vi "control.vi"() -> ()   [LabVIEW 2018]
uses:
  <vilib>/Analysis/Matrix/Datatypes/RealMatrix.ctl
  <vilib>/Analysis/Matrix/NI_Matrix.lvlib
panel:
  in  "stop":bool
  out "Matrix D":T1=[[-52.0, 0.0, 1.0], [-52.0, 0.0, 1.0], [0.0, 0.0, 1.0], [0.0, 0.0, 1.0]]
  out "m=D*v=(v1,v2,v3,v4)\n(desired)":T1
  in  "v=(v_r,v_t,Rw)'\n(desired)":T1
  # "OBS: v1,v2,v3,v4 conforme a numeração da placa-mãe"
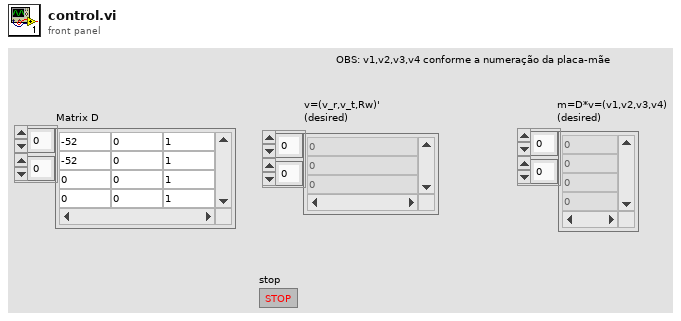
[diagram p1: front panel]
types:
  T1 = typedef "NI_Matrix.lvlib/RealMatrix.ctl" = dbl[][]
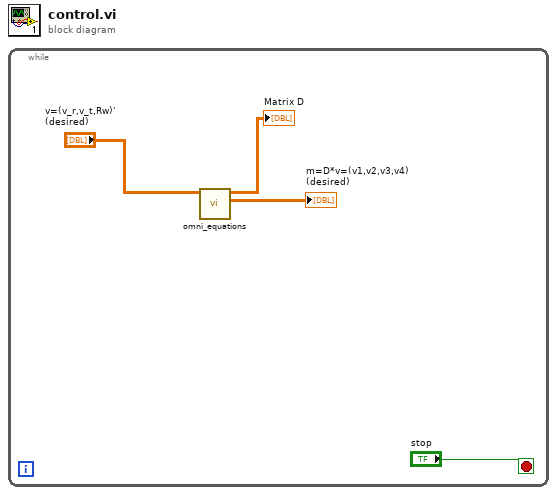
[diagram p0: block diagram]
diagram:
  n1 = while {
    stop <- "stop" stop-if-true
    n2 = call "omni_equations.vi"("v=(v_r,v_t,Rw)'"="v=(v_r,v_t,Rw)'\n(desired)") -> ("m=D*v=(v1,v2,v3,v4)"=→"m=D*v=(v1,v2,v3,v4)\n(desired)":T1, "Matrix D"=→"Matrix D":T1)  [unwired: 9 in]
  }
